vi "Agilent N6700 Series Read External Datalog.vi"() -> ()   [LabVIEW 2021]
doc: "Configures the external datalog then reads it from the instrument's buffer."
uses:
  <instrlib>/Agilent N6700 Series/Agilent N6700 Series.lvlib
panel:
  in  "error in":errorcluster {"code" format="%.0x"}
  out "error out":errorcluster {"code" format="%.0x"}
  out "External Log":string
  in  "Max Records":i32=10
  in  "Data Log Period":dbl=0.1
  in  "Data Log Type":i32(ring)=1 items=["Voltage"=1, "Current"=0]
  in  "Agilent SMU Channel":string="3"
  in  "Agilent SMU":refnum<visa-resource-name>
  # "Agilent N6700 DC Power Supply"
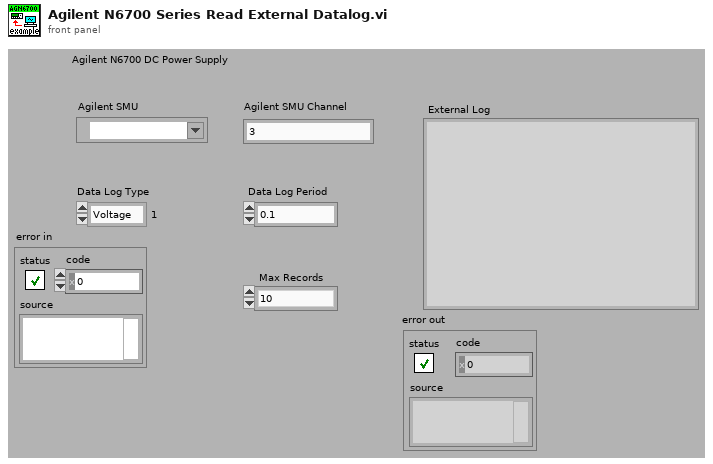
[diagram p1: front panel]
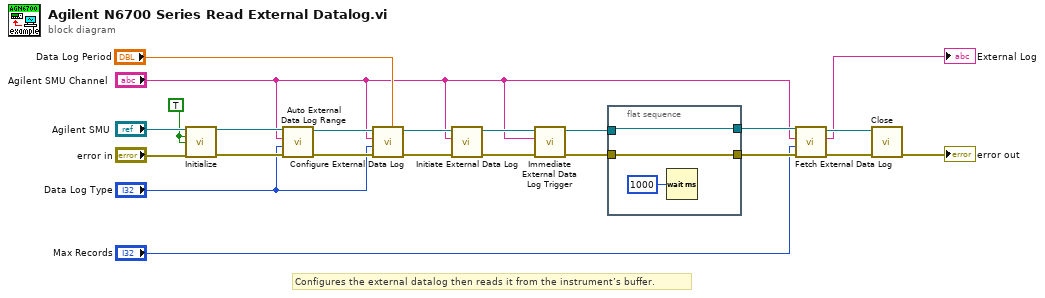
[diagram p0: block diagram]
diagram:
  w22 = TRUE ("Reset? (T: Yes)")
  # "Configures the external datalog then reads it from the instrument’s buffer."
  n1 = call <instrlib>:"Initialize.vi"("VISA resource name"="Agilent SMU", "ID Query? (T: Yes)"=w22, "Reset? (T: Yes)"=w22, "error in (no error)"="error in") -> ("VISA resource name out"=w21:refnum<visa-resource-name>, "error out"=w20:errorcluster)  [unwired: 10 in]
  n2 = call <instrlib>:"Auto External Data Log Range.vi"("error in (no error)"=w20, "External Data Log Type (1: Voltage)"="Data Log Type", "Channel Name (1)"="Agilent SMU Channel", "VISA resource name"=w21) -> ("error out"=w18:errorcluster, "VISA resource name out"=w19:refnum<visa-resource-name>)  [unwired: 6 in]
  n3 = call <instrlib>:"Configure External Data Log.vi"("External Data Log Period (0.1 s)"="Data Log Period", "error in (no error)"=w18, "External Data Log Type (1: Voltage)"="Data Log Type", "Channel Name (1)"="Agilent SMU Channel", "VISA resource name"=w19) -> ("error out"=w14:errorcluster, "VISA resource name out"=w15:refnum<visa-resource-name>)  [unwired: 5 in]
  n4 = call <instrlib>:"Initiate External Data Log.vi"("error in (no error)"=w14, "Channel Name (1)"="Agilent SMU Channel", "VISA resource name"=w15) -> ("error out"=w12:errorcluster, "VISA resource name out"=w13:refnum<visa-resource-name>)  [unwired: 7 in]
  n5 = call <instrlib>:"Immediate External Data Log Trigger.vi"("error in (no error)"=w12, "Channel Name (1)"="Agilent SMU Channel", "VISA resource name"=w13) -> ("error out"=w10:errorcluster, "VISA resource name out"=w11:refnum<visa-resource-name>)  [unwired: 7 in]
  n6 = flat-sequence {
    tunnel: w11 -> [w26]
    tunnel: [w26] -> w8
    tunnel: [w24] -> w9
    tunnel: w10 -> [w24]
    frame #0 {
      n7 = Wait (ms)(milliseconds to wait=u32 1000) -> ()  [unwired: 1 out]
    }
  }
  n8 = call <instrlib>:"Fetch External Data Log.vi"("error in (no error)"=w9, "Max Records (1)"="Max Records", "Channel Name (1)"="Agilent SMU Channel", "VISA resource name"=w8) -> ("error out"=w4:errorcluster, "External Log"=→"External Log":string, "VISA resource name out"=w5:refnum<visa-resource-name>)  [unwired: 5 in]
  n9 = call <instrlib>:"Close.vi"("VISA resource name"=w5, "error in (no error)"=w4) -> ("error out"=→"error out":errorcluster)  [unwired: 13 in]
